vi "BuildDrvInfo.vi"(5 "CameraDemo in":refnum<class "CameraDemo.lvclass">) -> (0 "CameraDemo out":refnum<class "CameraDemo.lvclass">, 2 "Lib Path":path, 3 "Class Name":string)   [LabVIEW 2020, in "CameraI2COUSB.lvlib" / "CameraDemo.lvclass"]
uses:
  CameraDemo.lvclass
panel:
  out "error out":errorcluster
  in  "error in (no error)":errorcluster
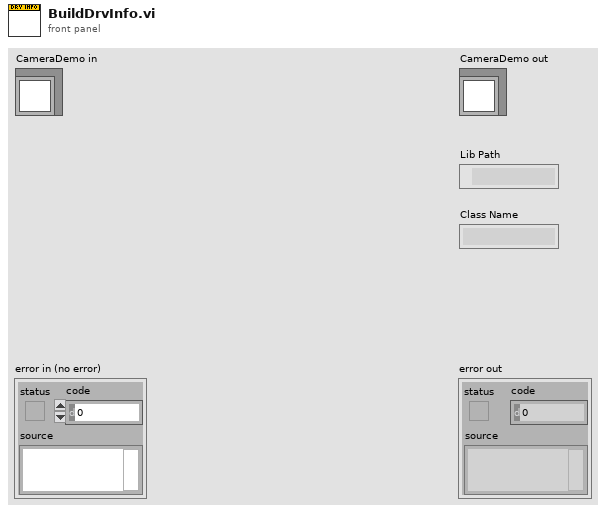
[diagram p1: front panel]
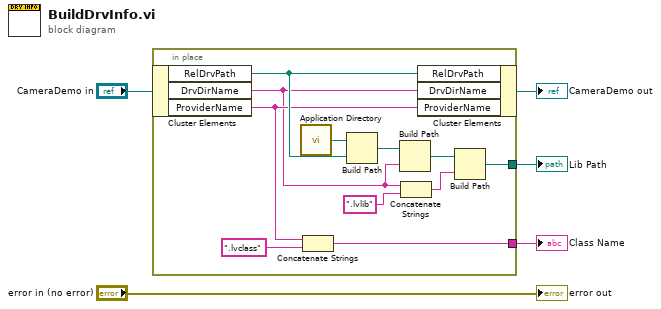
[diagram p0: block diagram]
diagram:
  n1 = in-place {
    in-place-border: [w11] -> w2
    in-place-border: [w7] -> w1
    n2 = in-place-cluster #1("CameraDemo in") -> ("RelDrvPath"=w9:path, "DrvDirName"=w6:string, "ProviderName"=w8:string)
    n3 = call <vilib>:"Application Directory.vi"() -> ("Application Directory"=w15:path)
    n4 = Concatenate Strings(w8, ".lvclass" ("y")) -> (w7:string)
    n5 = Build Path(base path=w15, name or relative path=w9) -> (appended path=w16:path)
    n6 = Build Path(base path=w16, name or relative path=w6) -> (appended path=w13:path)
    n7 = Concatenate Strings(w6, ".lvlib") -> (w12:string)
    n8 = in-place-cluster #1("RelDrvPath"=w9, "DrvDirName"=w6, "ProviderName"=w8) -> (→"CameraDemo out":refnum<class "CameraDemo.lvclass">)
    n9 = Build Path(base path=w13, name or relative path=w12) -> (appended path=w11:path)
  }
  "Class Name" <- w1
  "Lib Path" <- w2
  "error out" <- "error in (no error)"
